vi "GV.vi"() -> ()   [LabVIEW 2014]
panel:
  out "String 2":string
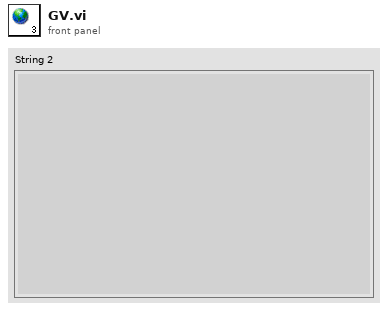
[diagram p1: front panel]
diagram:
